vi "GenerateSignal.vi"(1 "FolderParameters":T1, 2 "WaveParameters":T2, 3 "Number of Samples":i32, 4 "Sampling Rate":i32) -> (0 "Wave":dbl[](array[numeric]))   [LabVIEW 2017]
panel:
  # "Default unit for frontpanel is mm, s, V, deg"
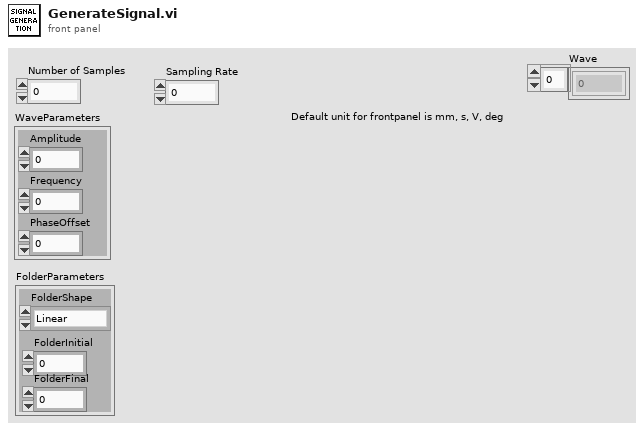
[diagram p1: front panel]
types:
  T1 = cluster{"FolderShape":enum16{"Linear", "Exponential"}, "FolderInitial":dbl, "FolderFinal":dbl}
  T2 = cluster{"Amplitude":dbl, "Frequency":i32, "PhaseOffset":dbl}
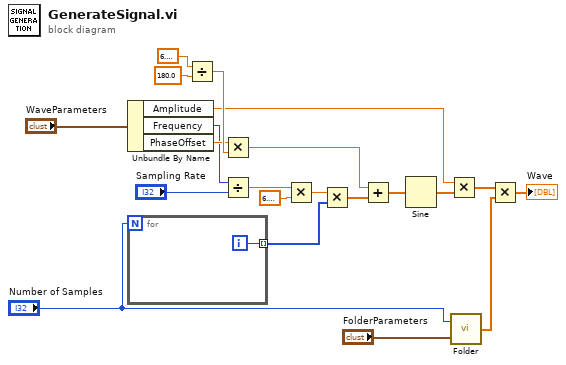
[diagram p0: block diagram]
diagram:
  n1 = Unbundle By Name("WaveParameters") -> ("Amplitude"=w11:dbl, "Frequency"=w4:i32, "PhaseOffset"=w10:dbl)
  n2 = for {
    N: "Number of Samples" -> [_]
    tunnel: [w22] -> w21 mode=indexing
    i -> [w22]
  }
  n3 = Divide(x=6.283185307179586, y=180.0) -> (x/y=w17:dbl)
  n4 = Multiply(x=w10, y=w17) -> (x*y=w14:dbl)
  n5 = Divide(x=w4, y="Sampling Rate") -> (x/y=w3:dbl)
  n6 = Multiply(x=w3, y=6.283185307179586) -> (x*y=w20:dbl)
  n7 = Multiply(x=w20, y=w21) -> (x*y=w18:dbl[])
  n8 = Add(x=w14, y=w18) -> (x+y=w7:dbl[])
  n9 = Sine(x=w7) -> (sin(x)=w6:dbl[])
  n10 = Multiply(x=w11, y=w6) -> (x*y=w1:dbl[])
  n11 = call "Folder.vi"("Parameters"="FolderParameters", "Number of Samples"="Number of Samples") -> ("Folder"=w2:dbl[])
  n12 = Multiply(x=w1, y=w2) -> (x*y=→"Wave":dbl[])
